vi "Abort.vi"(8 "error in (no error)":errorcluster, 11 "NI PXI Trigger in":refnum<class "NI PXI Trigger.lvclass">) -> (0 "error out":errorcluster, 3 "NI PXI Trigger out":refnum<class "NI PXI Trigger.lvclass">)   [LabVIEW 2020, in "NI DAQmx.lvlib" / "NI PXI Trigger.lvclass"]
uses:
  NI PXI Trigger.lvclass
  NI PXI Trigger.lvclass/NI PXI Trigger.ctl
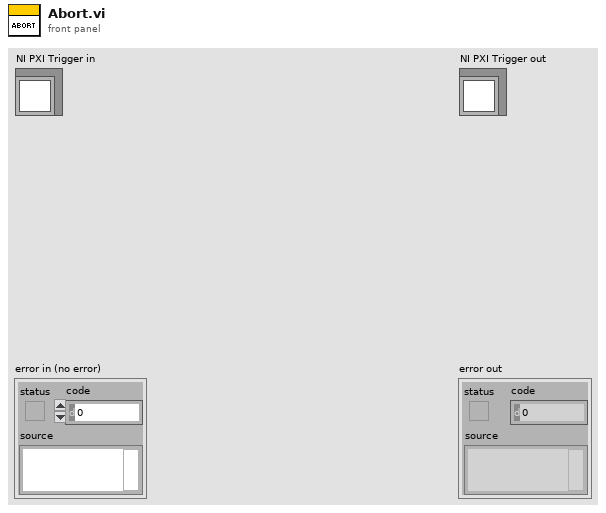
[diagram p1: front panel]
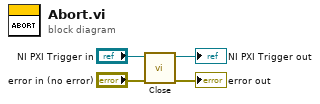
[diagram p0: block diagram]
diagram:
  n1 = call-dynamic "Close.vi"("error in (no error)"="error in (no error)", "NI PXI Trigger in"="NI PXI Trigger in") -> ("error out"=→"error out":errorcluster, "NI PXI Trigger out"=→"NI PXI Trigger out":refnum<class "NI PXI Trigger.lvclass">)  [unwired: 8 in]
